vi "点是否在合法范围.vi"(8 "错误输入（无错误）":errorcluster, 10 "点":T1, 11 "Table输入":refnum<vi>) -> (0 "错误输出":errorcluster, 2 "是否在范围":bool, 3 "引用输出":refnum<vi>, 4 "列":i32, 6 "行":i32)   [LabVIEW 2014, in "表格.lvlib"]
uses:
  <vilib>/Utility/miscctls.llb/LVPositionTypeDef.ctl
  <vilib>/Utility/miscctls.llb/LVRowAndColumnTypeDef.ctl
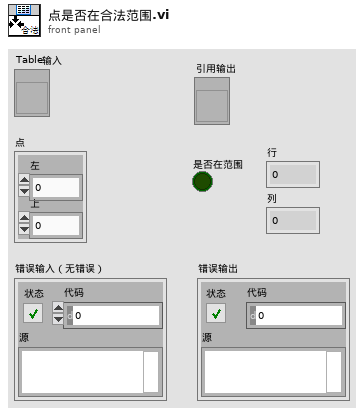
[diagram p1: front panel]
types:
  T1 = typedef "LVPositionTypeDef.ctl" = cluster{"Left":i32, "Top":i32}
  T2 = typedef "LVRowAndColumnTypeDef.ctl" = cluster{"Row":i32, "Column":i32}
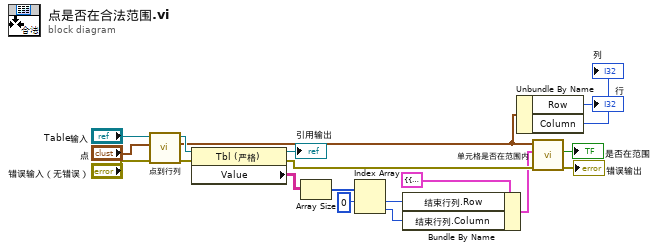
[diagram p0: block diagram]
diagram:
  n1 = call "点到行列.vi"("错误输入（无错误）"="错误输入（无错误）", "点"="点", "引用"="Table输入") -> ("错误输出"=w9:errorcluster, "单元格位置"=w3:T2, "引用输出"=w8:refnum<vi>)  [unwired: 6 in]
  n2 = property class="Tbl (严格)"(reference=w8, error in=w9) -> (reference out=→"引用输出":refnum<vi>, error out=w18:errorcluster, "Value"=w10:string[][])
  n3 = Array Size(array=w10) -> (size(s)=w12:i32[])
  n4 = Index Array(array=w12, index #1=0 ("索引")) -> (element #1=w14:i32, element #2=w15:i32)  [unwired: 1 in]
  n5 = Bundle By Name(cluster=cluster{"起始行列":T2, "结束行列":T2} {"起始行列"={"Row"=0, "Column"=0}, "结束行列"={"Row"=0, "Column"=0}} ("行列范围"), "结束行列.Row"=w14, "结束行列.Column"=w15) -> (w16:cluster{"起始行列":T2, "结束行列":T2})
  n6 = Unbundle By Name(w3) -> ("Row"=→"行":i32, "Column"=→"列":i32)
  n7 = call "单元格是否在范围内.vi"("error in (no error)"=w18, "行列范围"=w16, "单元格位置"=w3) -> ("error out"=→"错误输出":errorcluster, "是否在范围"=→"是否在范围":bool)  [unwired: 6 in, 1 out]
